vi "xijk_remove_filenames.vi"(1 "chemin":path) -> (0 "output":string)   [LabVIEW 2009]
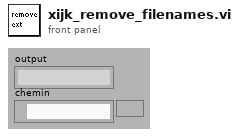
[diagram p1: front panel]
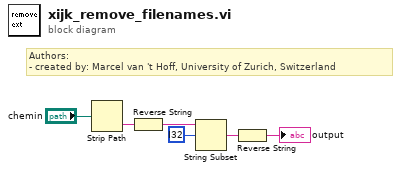
[diagram p0: block diagram]
diagram:
  # "Authors: \n- created by: Marcel van 't Hoff, University of Zurich, Switzerland"
  n1 = Strip Path(path="chemin") -> (name=w1:string)  [unwired: 1 out]
  n2 = Reverse String(1:w1) -> (0:w6:string)
  n3 = String Subset(string=w6, offset (0)=i32 ?) -> (substring=w4:string)  [unwired: 1 out]
  n4 = Reverse String(1:w4) -> (0:→"output":string)
